vi "Calculate Counter Value.vi"(9 "Overrides":dbl[](array[numeric]), 10 "Frame.Data in":dbl[](array[numeric]), 11 "Counter Configuration in":T1) -> (1 "Counter Value":dbl, 2 "Frame.Data out":dbl[](array[numeric]), 3 "Counter Configuration out":T1)   [LabVIEW 2019, in "Protection and Counter Support Engine.lvlib"]
uses:
  Protection and Counter Support Engine.lvlib
  Shared/Types/Exported Counter Settings.ctl
  Shared/Protection and Counter Support Shared.lvlib
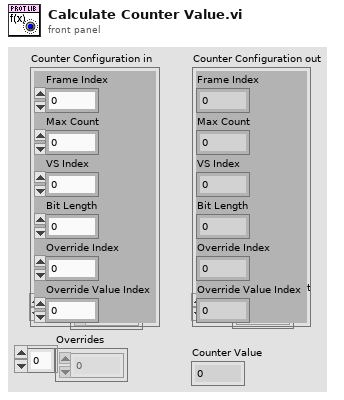
[diagram p1: front panel]
types:
  T1 = typedef "Protection and Counter Support Shared.lvlib/Exported Counter Settings.ctl" = cluster{"Frame Index":i32, "Max Count":dbl, "VS Index":i32, "Bit Length":i64, "Override Index":i32, "Override Value Index":i32}
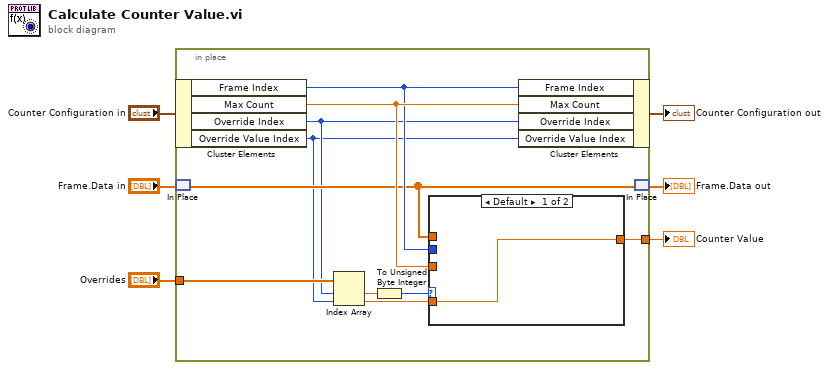
[diagram p0: block diagram]
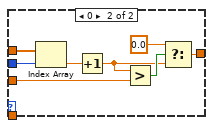
[diagram p2: hidden frame]
diagram:
  n1 = in-place {
    in-place-border: [w16] -> w2
    in-place-border: "Overrides" -> [w12]
    n2 = in-place-cluster #1("Counter Configuration in") -> ("Frame Index"=w14:i32, "Max Count"=w15:dbl, "Override Index"=w11:i32, "Override Value Index"=w10:i32)
    n3 = in-place-match #2("Frame.Data in") -> (w13:dbl[])
    n4 = Index Array(array=w12, index #1=w11, index #2=w10) -> (element #1=w9:dbl, element #2=w7:dbl)
    n5 = To Unsigned Byte Integer(number=w9) -> (unsigned 8bit integer=w8:u8)
    n6 = case shown="Default" w8 {
      tunnel: [w17 w21] -> w16
      tunnel: w15 -> [_ w20]
      tunnel: w14 -> [_ w19]
      tunnel: w13 -> [_ w18]
      tunnel: w7 -> [w17 _]
      frame Default {
      }
      frame 0 {
        n7 = Index Array(array=w18, index=w19) -> (element=w23:dbl)
        n8 = Increment(x=w23) -> (x+1=w22:dbl)
        n9 = Greater?(x=w22, y=w20) -> (0:w25:bool)
        n10 = Select(t=0.0, s=w25, f=w22) -> (s? t:f=w21:dbl)
      }
    }
    n11 = in-place-cluster #1("Frame Index"=w14, "Max Count"=w15, "Override Index"=w11, "Override Value Index"=w10) -> (→"Counter Configuration out":T1)
    n12 = in-place-match #2(w13) -> (→"Frame.Data out":dbl[])
  }
  "Counter Value" <- w2
